vi "Read(Y)Trace.vi"(8 "error in (no error)":errorcluster, 11 "SpecAnBase in":refnum<class "SpecAnBase.lvclass">) -> (0 "error out":errorcluster, 3 "SpecAnBase out":refnum<class "SpecAnBase.lvclass">)   [LabVIEW 2014, in "SpecAnPlugins.lvlib" / "SpecAnBase.lvclass"]
doc: "This function initiates a signal acquisition based on the present instrument configuration. It then waits for the acquisition to complete, and returns the trace as an array of amplitude values. The amplitude array returns data that represent the amplitude of the signals obtained by sweeping from the start frequency to the stop frequency (in frequency domain, in time domain the amplitude array is ordered from beginning of sweep to end). The Amplitude Units attribute determines the units of the points in the amplitude array. This function resets the sweep count.\n\nIf the spectrum analyzer did not complete the acquisition within the time period the user specified with the MaxTime parameter, the function returns the Max Time Exceeded error."
uses:
  SpecAnBase.lvclass
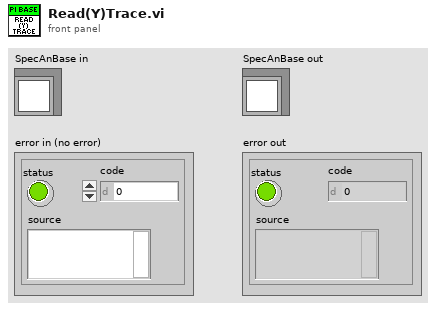
[diagram p1: front panel]
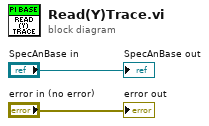
[diagram p0: block diagram]
diagram:
  "error out" <- "error in (no error)"
  "SpecAnBase out" <- "SpecAnBase in"
